vi "RW UDVs.vi"(7 "R/W Case":T2, 8 "error in (no error)":errorcluster, 10 "Async in":T1, 11 "FPGA in":T3[](array[typedef]) {"UDVs"."To FPGA"."VS ref" format="%.0x"; "UDVs"."From FPGA"."VS ref" format="%.0x"; "VS ref" format="%.0x"; "Output Data"."BD Refs"."Data Reference" format="%.0x"; "Input Data"."BD Refs"."Data Reference" format="%.0x"}) -> (0 "error out":errorcluster, 2 "Async out":T1, 3 "FPGA out":T3[](array[typedef]) {"UDVs"."To FPGA"."VS ref" format="%.0x"; "UDVs"."From FPGA"."VS ref" format="%.0x"; "VS ref" format="%.0x"; "Output Data"."BD Refs"."Data Reference" format="%.0x"; "Input Data"."BD Refs"."Data Reference" format="%.0x"})   [LabVIEW 2016, in "Scan Engine Custom Device.lvlib"]
uses:
  Scan Engine Custom Device.lvlib
  Type Defs/FPGA Data.ctl
  <vilib>/NI Veristand/Custom Device API/Custom Device Item Ref.ctl
  Type Defs/Input Data.ctl
  <vilib>/NI Veristand/Custom Device API/Block Data Reference.ctl
  <vilib>/NI Veristand/Custom Device API/Data Reference.ctl
  Type Defs/Output Data.ctl
  Type Defs/UDV Data.ctl
  Type Defs/UDV Data Type.ctl
  Type Defs/FXP Config.ctl
  Type Defs/RW Case.ctl
  Type Defs/Async Data.ctl
  Type Defs/Async Status.ctl
  Type Defs/Async State.ctl
  Type Defs/Async Command.ctl
  Scanned Read - UDV.vi
  <vilib>/NI Veristand/Custom Device API/NI VeriStand - Set Channel Values by Block Data Reference.vi
  Scanned Write - UDV.vi
  <vilib>/NI Veristand/Custom Device API/NI VeriStand - Get Channel Values by Block Data Reference.vi
  <vilib>/NI Veristand/Custom Device API/Global Data Refs.vi
  <vilib>/NI Veristand/Custom Device API/Custom Device API.lvlib
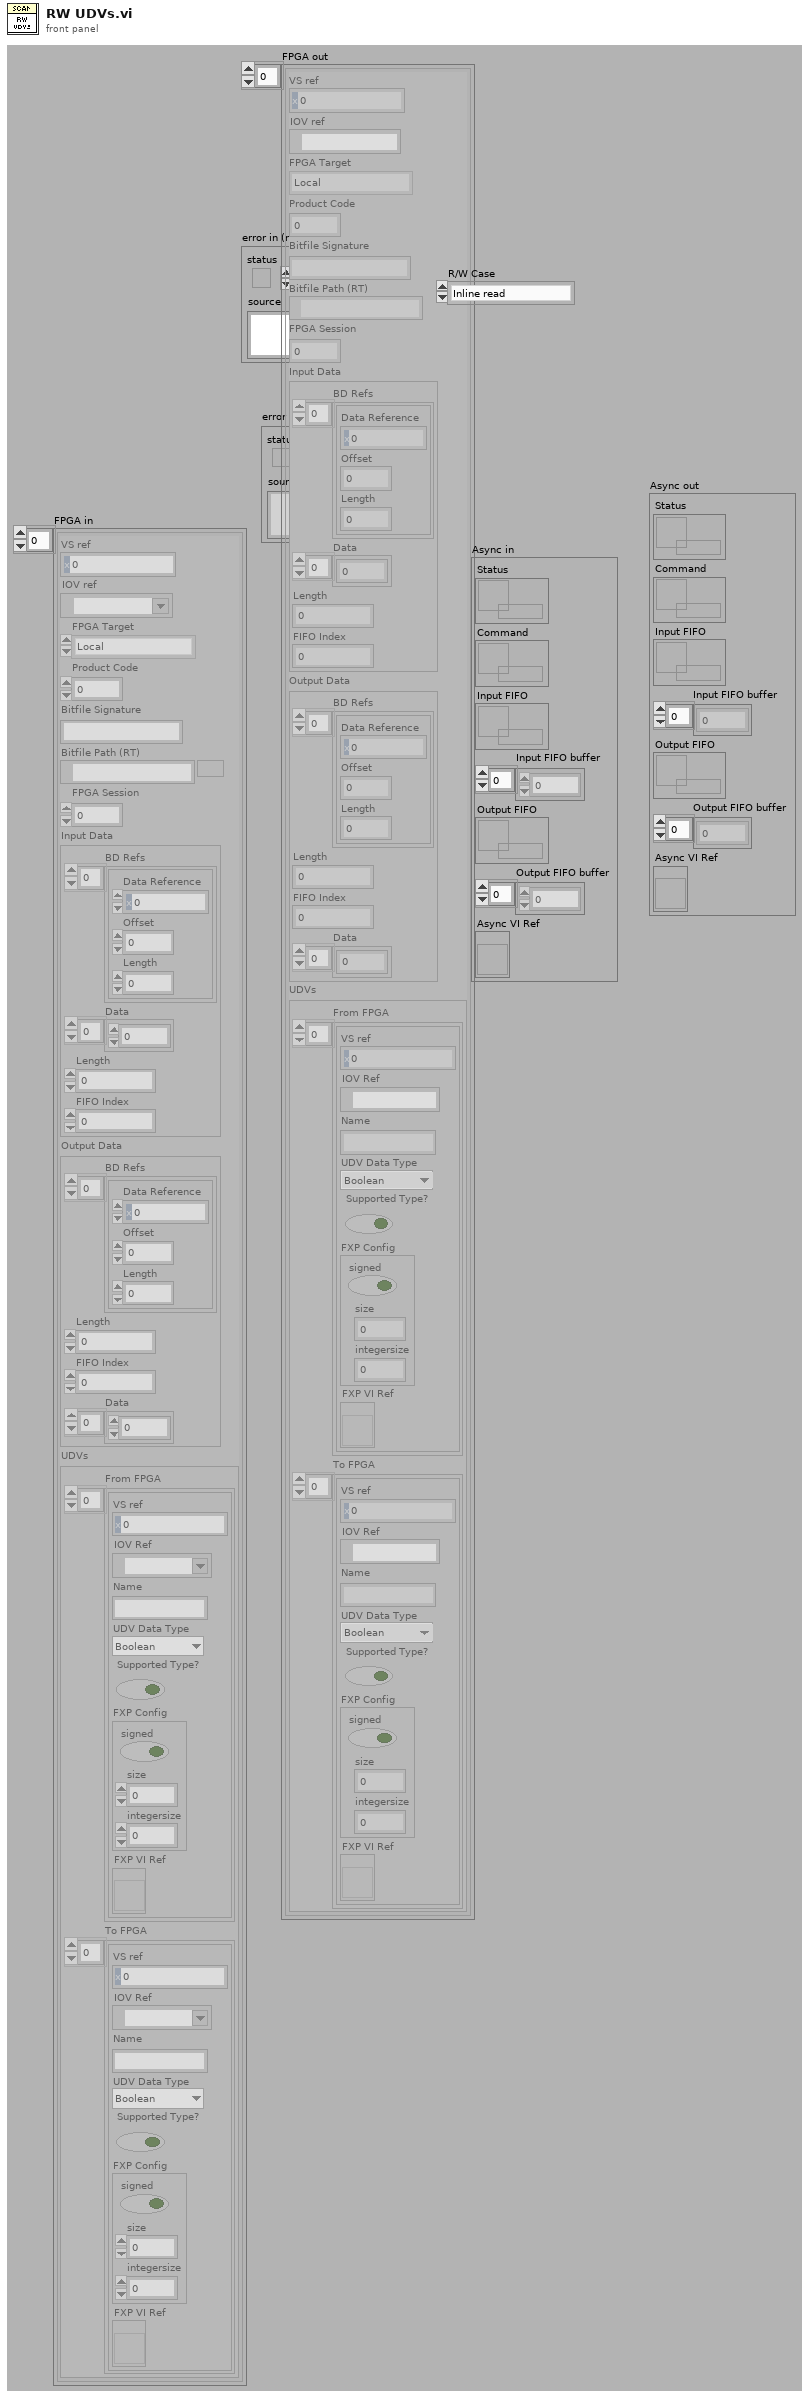
[diagram p1: front panel]
types:
  T1 = typedef "Scan Engine Custom Device.lvlib/Async Data.ctl" = cluster{"Status":refnum<queue>, "Command":refnum<queue>, "Input FIFO":refnum<k33>, "Input FIFO buffer":dbl[], "Output FIFO":refnum<k33>, "Output FIFO buffer":dbl[], "Async VI Ref":refnum<vi>}
  T2 = typedef "Scan Engine Custom Device.lvlib/RW Case.ctl" = enum16{"Inline read", "Inline write", "Async - Inline loop read", "Async - Inline loop write", "Async loop (read/write)"}
  T3 = typedef "Scan Engine Custom Device.lvlib/FPGA Data.ctl" = cluster{"VS ref":T4, "IOV ref":refnum<k21>, "FPGA Target":enum16{"Local", "EtherCAT"}, "Product Code":u32, "Bitfile Signature":string, "Bitfile Path (RT)":path, "FPGA Session":u32, "Input Data":T5, "Output Data":T8, "UDVs":cluster{"From FPGA":T9[], "To FPGA":T9[]}}
  T4 = typedef "Custom Device API.lvlib/Custom Device Item Ref.ctl" = u64
  T5 = typedef "Scan Engine Custom Device.lvlib/Input Data.ctl" = cluster{"BD Refs":T6[], "Data":dbl[], "Length":i32, "FIFO Index":i32}
  T6 = typedef "Custom Device API.lvlib/Block Data Reference.ctl" = cluster{"Data Reference":T7, "Offset":u64, "Length":u64}
  T7 = typedef "Custom Device API.lvlib/Data Reference.ctl" = i32
  T8 = typedef "Scan Engine Custom Device.lvlib/Output Data.ctl" = cluster{"BD Refs":T6[], "Length":i32, "FIFO Index":i32, "Data":dbl[]}
  T9 = typedef "Scan Engine Custom Device.lvlib/UDV Data.ctl" = cluster{"VS ref":T4, "IOV Ref":refnum<k21>, "Name":string, "UDV Data Type":T10, "Supported Type?":bool, "FXP Config":T11, "FXP VI Ref":refnum<vi>}
  T10 = typedef "Scan Engine Custom Device.lvlib/UDV Data Type.ctl" = enum16{"Boolean", "Fixed Point", "Int8", "Int16", "Int32", "Int64", "U32 Bit Field", "UInt8", "UInt16", "UInt32", "UInt64", "Other"}
  T11 = typedef "Scan Engine Custom Device.lvlib/FXP Config.ctl" = cluster{"signed":bool, "size":u32, "integersize":i32}
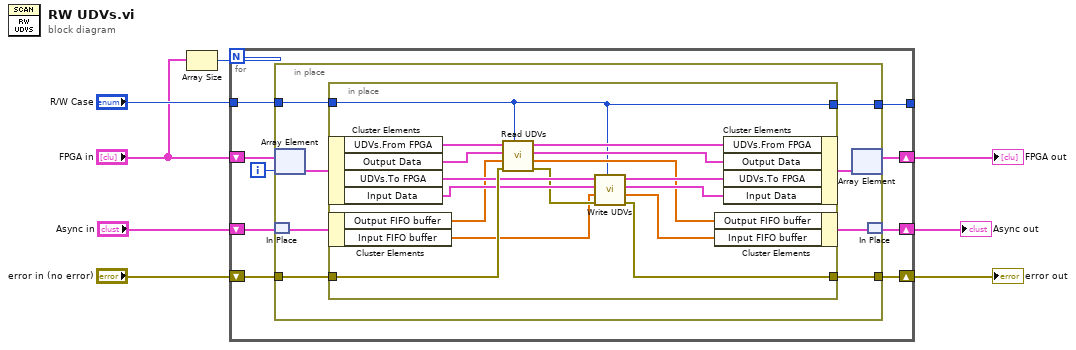
[diagram p0: block diagram]
diagram:
  n1 = Array Size(array="FPGA in") -> (size(s)=w5:i32)
  n2 = for {
    N: w5 -> [_]
    shift-right: [w15] -> w6
    shift-left: "FPGA in" -> [w17]
    shift-right: [w12] -> w7
    shift-left: "error in (no error)" -> [w14]
    tunnel: "R/W Case" -> [w13]
    shift-right: [w10] -> w3
    shift-left: "Async in" -> [w11]
    tunnel: [w9] -> _
    i -> [w16]
    n3 = in-place {
      in-place-border: w14 -> [w23]
      in-place-border: w13 -> [w22]
      in-place-border: [w21] -> w12
      in-place-border: [w18] -> w9
      n4 = in-place-array #1(w17, w16) -> (w25:T3)
      n5 = in-place-match #2(w11) -> (w20:T1)
      n6 = in-place {
        in-place-border: w23 -> [w37]
        in-place-border: w22 -> [w26]
        in-place-border: [w32] -> w21
        in-place-border: [w26] -> w18
        n7 = in-place-cluster #3(w25) -> ("UDVs.From FPGA"=w41:T9[], "Output Data"=w40:T8, "UDVs.To FPGA"=w36:T9[], "Input Data"=w34:T5)
        n8 = in-place-cluster #4(w20) -> ("Output FIFO buffer"=w30:dbl[], "Input FIFO buffer"=w28:dbl[])
        n9 = call "Read UDVs.vi"("R/W Case"=w26, "error in (no error)"=w37, "Output FIFO buffer in"=w30, "Output Data in"=w40, "UDVs in"=w41) -> ("error out"=w33:errorcluster, "Output FIFO buffer out"=w29:dbl[], "Output Data out"=w38:T8, "UDVs out"=w39:T9[])  [unwired: 3 in]
        n10 = call "Write UDVs.vi"("R/W Case"=w26, "error in (no error)"=w33, "Input FIFO buffer in"=w28, "Input Data in"=w34, "UDVs in"=w36) -> ("error out"=w32:errorcluster, "Input FIFO buffer out"=w27:dbl[], "Input Data out"=w31:T5, "UDVs out"=w35:T9[])  [unwired: 3 in]
        n11 = in-place-cluster #4("Output FIFO buffer"=w29, "Input FIFO buffer"=w27) -> (w19:T1)
        n12 = in-place-cluster #3("UDVs.From FPGA"=w39, "Output Data"=w38, "UDVs.To FPGA"=w35, "Input Data"=w31) -> (w24:T3)
      }
      n13 = in-place-array #1(w24) -> (w15:T3[])  [unwired: 1 out]
      n14 = in-place-match #2(w19) -> (w10:T1)
    }
  }
  "error out" <- w7
  "FPGA out" <- w6
  "Async out" <- w3
